vi "instantiate_simple_qa_dynamic.vi"(0 "vectorestore":refnum<class "abstract_vector_base.lvclass">, 1 "skip_loading_data":bool, 5 "collection_name":string, 7 "chat_model":refnum<class "abstract_llm_base.lvclass">, 9 "embedding_model":refnum<class "abstract_llm_base.lvclass">, 11 "error in (no error)":errorcluster, 12 "sources":string[](array[string])) -> (4 "agent_webpage_qa out":refnum<class "agent_simple_qa_dynamic.lvclass">, 15 "error out":errorcluster)   [LabVIEW 2020, in "agent_simple_qa_dynamic.lvclass"]
uses:
  agent_simple_qa_dynamic.lvclass
  D:/Personal/LabVIEW LLMs/src/agent/agent_simple_qa/agent_simple_qa.lvclass
  models/abstract_llm_base/abstract_llm_base.lvclass
  vectorstore/abstract_vector_base/abstract_vector_base.lvclass
  data_source/datasource_text_file/datasource_text_file.lvclass
  D:/Personal/LabVIEW LLMs/src/data_source/abstract_datasource_base/abstract_datasource_base.lvclass
  data_source/datasource_webpage/datasource_webpage.lvclass
  data_source/datasource_pdf/datasource_pdf.lvclass
  data_destination/destination_vectorstore/destination_vectorstore.lvclass
  D:/Personal/LabVIEW LLMs/src/data_destination/abstract_datadestination_base/abstract_datadestination_base.lvclass
  data_processor/chunk_character_splitter/chunk_character_splitter.lvclass
  D:/Personal/LabVIEW LLMs/src/data_processor/abstract_dataprocessing_base/abstract_dataprocessing_base.lvclass
  data_processor/embed_nodes/embed_nodes.lvclass
  data_pipeline/data_simple_pipeline/data_simple_pipeline.lvclass
  data_processor/abstract_dataprocessing_base/abstract_dataprocessing_base.lvclass
  data_source/abstract_datasource_base/abstract_datasource_base.lvclass
  agent_simple_qa/agent_simple_qa.lvclass
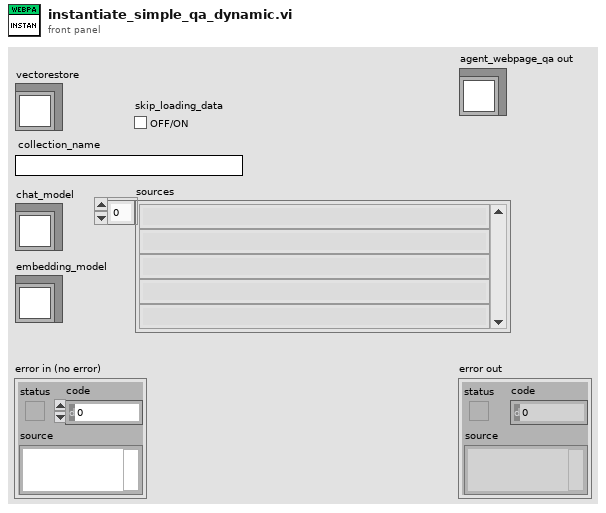
[diagram p1: front panel]
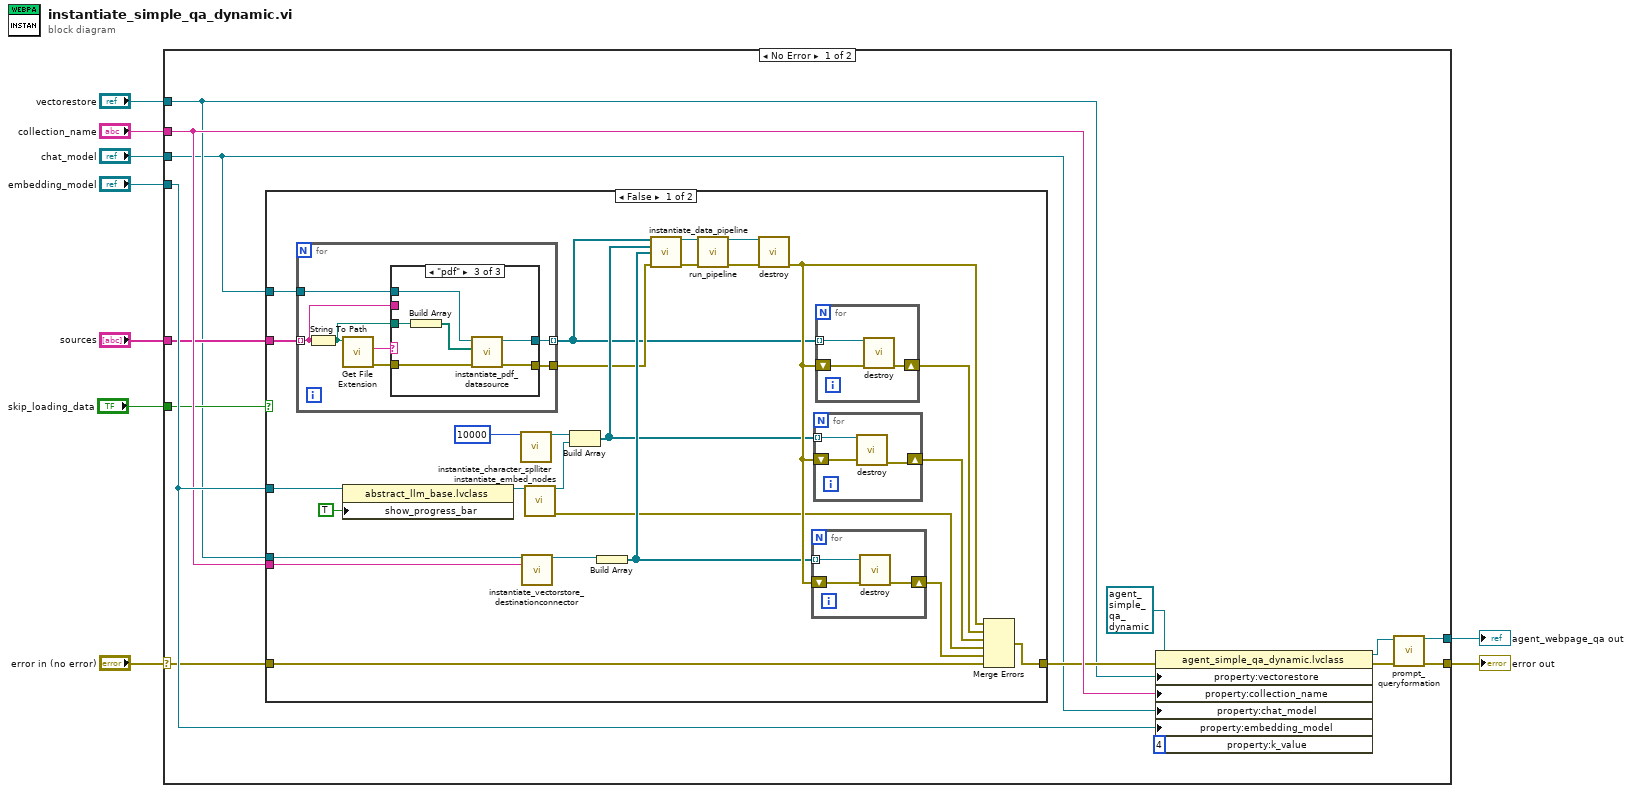
[diagram p0: block diagram]
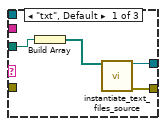
[diagram p2: hidden frame]
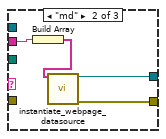
[diagram p3: hidden frame]
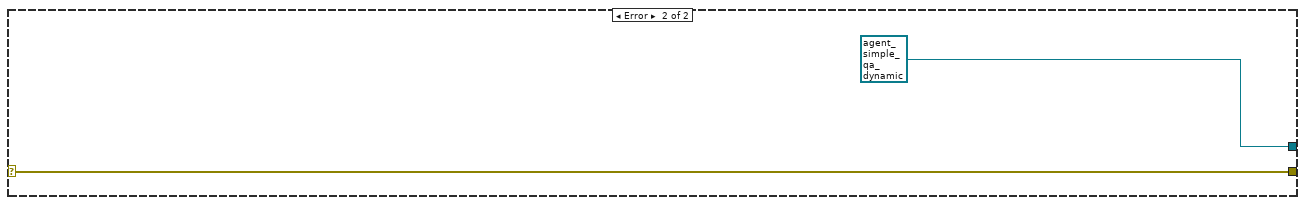
[diagram p5: hidden frame]
diagram:
  n1 = case shown="No Error" "error in (no error)" {
    selector: "error in (no error)" -> [w15 w82]
    tunnel: [w19 w82] -> w8
    tunnel: "vectorestore" -> [w11 _]
    tunnel: "collection_name" -> [w16 _]
    tunnel: "chat_model" -> [w10 _]
    tunnel: "embedding_model" -> [w17 _]
    tunnel: [w18 refnum<class "agent_simple_qa_dynamic.lvclass"> refnum ("agent_webpage_qa out")] -> w3
    tunnel: "sources" -> [w13 _]
    tunnel: "skip_loading_data" -> [w12 _]
    frame No Error {
      n2 = case shown="False" w12 {
        tunnel: w17 -> [w36 _]
        tunnel: w11 -> [w33 _]
        tunnel: w16 -> [w32 _]
        tunnel: w15 -> [w31 w80]
        tunnel: [w30 w80] -> w14
        tunnel: w13 -> [w27 _]
        tunnel: w10 -> [w24 _]
        frame False {
          n3 = for {
            tunnel: w27 -> [w53] mode=indexing
            tunnel: [w56] -> w26
            tunnel: [w55] -> w25 mode=indexing
            tunnel: w24 -> [w50]
            n4 = String To Path(string=w53) -> (path=w51:path)
            n5 = call <vilib>:"Get File Extension.vi"("file"=w51) -> ("error out"=w52:errorcluster, "lowercase file extension"=w54:string)  [unwired: 6 in, 3 out]
            n6 = case shown="\"pdf\"" w54 {
              tunnel: [w59 w64 w69] -> w56
              tunnel: [w60 w63 w65] -> w55
              tunnel: w53 -> [_ w62 _]
              tunnel: w52 -> [_ _ w70]
              tunnel: w51 -> [w58 _ w68]
              tunnel: w50 -> [_ _ w66]
              frame "txt", Default {
                n7 = Build Array(w58) -> (w57:path[])
                n8 = call "instantiate_text_files_source.vi"("text files"=w57) -> ("datasource_text_file out"=w60:refnum<class "datasource_text_file.lvclass">, "error out"=w59:errorcluster)  [unwired: 13 in]
              }
              frame "md" {
                n9 = Build Array(w62) -> (w61:string[])
                n10 = call "instantiate_webpage_datasource.vi"("webpages"=w61) -> ("datasource_webpage out"=w63:refnum<class "datasource_webpage.lvclass">, "error out"=w64:errorcluster)  [unwired: 13 in]
              }
              frame "pdf" {
                n11 = Build Array(w68) -> (w67:path[])
                n12 = call "instantiate_pdf_datasource.vi"("error in (no error)"=w70, "file_list"=w67, "llm"=w66) -> ("error out"=w69:errorcluster, "datasource_pdf out"=w65:refnum<class "datasource_pdf.lvclass">)  [unwired: 7 in]
              }
            }
          }
          n13 = property class="abstract_llm_base.lvclass"(reference=w36, "show_progress_bar"=TRUE) -> (reference out=w29:refnum<class "abstract_llm_base.lvclass">)  [unwired: 1 in, 1 out]
          n14 = call "instantiate_character_splliter.vi"("max_character_length"=u32 10000) -> ("chunk_character_splitter out"=w42:refnum<class "chunk_character_splitter.lvclass">)  [unwired: 13 in, 1 out]
          n15 = call "instantiate_vectorstore_destinationconnector.vi"("abstract_vector_base"=w33, "store_id"=w32) -> ("destination_vectorstore out"=w46:refnum<class "destination_vectorstore.lvclass">)  [unwired: 12 in, 1 out]
          n16 = call "instantiate_embed_nodes.vi"("abstract_llm_embedding"=w29) -> ("embed_nodes out"=w43:refnum<class "embed_nodes.lvclass">, "error out"=w35:errorcluster)  [unwired: 13 in]
          n17 = Build Array(w42, w43) -> (w44:refnum<class "abstract_dataprocessing_base.lvclass">[])
          n18 = Build Array(w46) -> (w47:refnum<class "destination_vectorstore.lvclass">[])
          n19 = call "instantiate_data_pipeline.vi"("sources"=w25, "processing steps"=w44, "destinations"=w47, "error in (no error)"=w26) -> ("data_simple_pipeline out"=w38:refnum<class "data_simple_pipeline.lvclass">, "error out"=w39:errorcluster)  [unwired: 10 in]
          n20 = call-dynamic "run_pipeline.vi"("data_simple_pipeline in"=w38, "error in (no error)"=w39) -> ("data_simple_pipeline out"=w40:refnum<class "data_simple_pipeline.lvclass">, "error out"=w41:errorcluster)  [unwired: 12 in]
          n21 = call-dynamic "destroy.vi"("data_simple_pipeline in"=w40, "error in (no error)"=w41) -> ("error out"=w49:errorcluster)  [unwired: 12 in, 1 out]
          n22 = for {
            shift-right: [w73] -> w34
            shift-left: w49 -> [w72]
            tunnel: w47 -> [w71] mode=indexing
            n23 = call-dynamic "destroy.vi"("abstract_datadestination_base in"=w71, "error in (no error)"=w72) -> ("error out"=w73:errorcluster)  [unwired: 12 in, 1 out]
          }
          n24 = for {
            tunnel: w44 -> [w76] mode=indexing
            shift-right: [w74] -> w45
            shift-left: w49 -> [w75]
            n25 = call-dynamic "destroy.vi"("abstract_dataprocessing_base in"=w76, "error in (no error)"=w75) -> ("error out"=w74:errorcluster)  [unwired: 12 in, 1 out]
          }
          n26 = for {
            tunnel: w25 -> [w79] mode=indexing
            shift-right: [w77] -> w48
            shift-left: w49 -> [w78]
            n27 = call-dynamic "destroy.vi"("abstract_datasource_base in"=w79, "error in (no error)"=w78) -> ("error out"=w77:errorcluster)  [unwired: 12 in, 1 out]
          }
          n28 = Merge Errors(w49, w48, w45, w35, w34, w31) -> (w30:errorcluster)
        }
        frame True {
        }
      }
      n29 = property class="agent_simple_qa_dynamic.lvclass"(reference=refnum<class "agent_simple_qa_dynamic.lvclass"> refnum ("agent_webpage_qa out"), error in=w14, "property:vectorestore"=w11, "property:collection_name"=w16, "property:chat_model"=w10, "property:embedding_model"=w17, "property:k_value"=u32 4 ("k_value")) -> (reference out=w20:refnum<class "agent_simple_qa_dynamic.lvclass">, error out=w21:errorcluster)
      n30 = call "prompt_queryformation.vi"("error in (no error)"=w21, "agent_simple_qa in"=w20) -> ("error out"=w19:errorcluster, "agent_simple_qa out"=w18:refnum<class "agent_simple_qa_dynamic.lvclass">)  [unwired: 8 in]
    }
    frame Error {
    }
  }
  "error out" <- w8
  "agent_webpage_qa out" <- w3
